vi "Partie 1.vi"() -> ()   [LabVIEW 2020]
uses:
  <instrlib>/Agilent 34401/Public/Data/Read (Multiple Points).vi
  <instrlib>/Agilent 2000 3000 X-Series/Public/Data/Read Measurement (Current Value).vi
  <instrlib>/Agilent 34401/Agilent 34401.lvlib
  <instrlib>/Agilent 2000 3000 X-Series/Agilent 2000 3000 X-Series.lvlib
panel:
  out "Nom du fichier":string
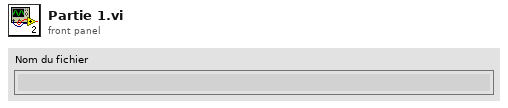
[diagram p1: front panel]
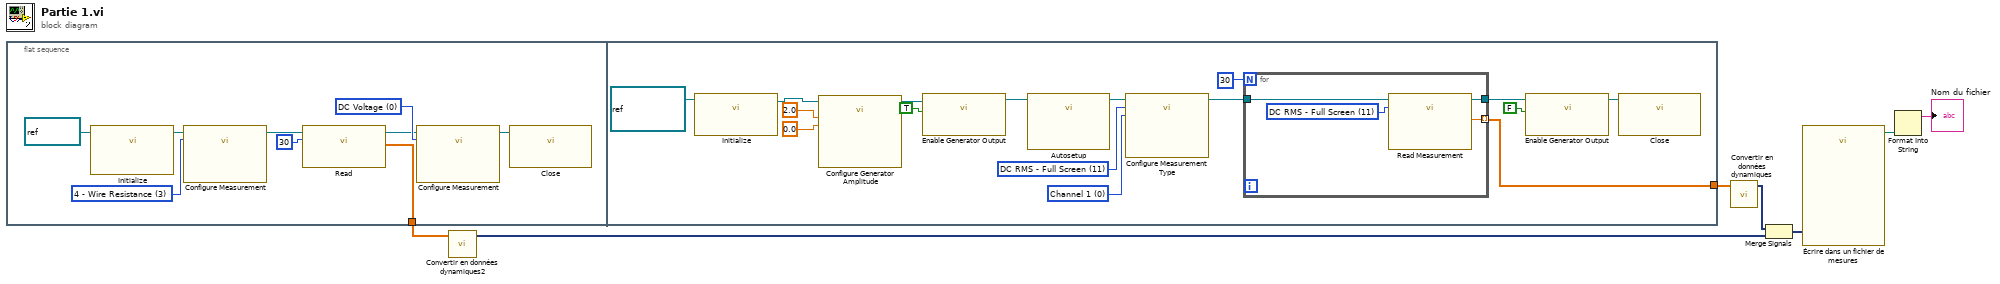
[diagram p0: block diagram]
diagram:
  n1 = flat-sequence {
    tunnel: [w10] -> w4
    tunnel: [w22] -> w7
    frame #0 {
      w16 = u16 0 items=["DC Voltage", "AC Voltage", "2 - Wire Resistance", "4 - Wire Resistance", "DC Current", "AC Current", "Frequency", "Period", "Continuity", "Diode Checking", "VDC:VDC Ratio", "Temperature", "Capacitance"] ("Function (0: DC Voltage)")
      w14 = u16 3 items=["DC Voltage", "AC Voltage", "2 - Wire Resistance", "4 - Wire Resistance", "DC Current", "AC Current", "Frequency", "Period", "Continuity", "Diode Checking", "VDC:VDC Ratio", "Temperature", "Capacitance"] ("Function (0: DC Voltage)")
      n2 = call <instrlib>:"Initialize.vi"("VISA resource name"=refnum<visa-resource-name> "GPIB0::22::INSTR") -> ("VISA resource name out"=w8:refnum<visa-resource-name>)  [unwired: 9 in, 1 out]
      n3 = call <instrlib>:"Configure Measurement.vi"("Function (0: DC Voltage)"=w14, "VISA resource name"=w8) -> ("VISA resource name out"=w13:refnum<visa-resource-name>)  [unwired: 8 in, 1 out]
      n4 = call-poly <instrlib>:"Read.vi"("Sample Count (1)"=30, "VISA resource name"=w13) -> ("Measurements"=w10:dbl[], "VISA resource name out"=w12:refnum<visa-resource-name>)  [unwired: 7 in, 1 out]
      n5 = call <instrlib>:"Configure Measurement.vi"("Function (0: DC Voltage)"=w16, "VISA resource name"=w12) -> ("VISA resource name out"=w9:refnum<visa-resource-name>)  [unwired: 8 in, 1 out]
      n6 = call <instrlib>:"Close.vi"("VISA resource name"=w9) -> ()  [unwired: 10 in, 1 out]
    }
    frame #1 {
      w29 = 0 items=["Channel 1"=0, "Channel 2"=1, "Channel 3"=2, "Channel 4"=3, "Waveform Memory 1"=5, "Waveform Memory 2"=6, "Serial Bus 1"=7, "Serial Bus 2"=8, "Digital Bus Low"=9, "Digital Bus High "=10, "Digital Bus 1"=11, "Digital Bus 2"=12, "D0"=13, "D1"=14, "D2"=15, "D3"=16, "D4"=17, "D5"=18, "D6"=19, "D7"=20, "D8"=21, "D9"=22, "D10"=23, "D11"=24, "D12"=25, "D13"=26, "D14"=27, "D15"=28, "External"=29, "Function 1"=32, "Function 2"=33, "Function 3"=34, "Function 4"=35, "Math 1"=36, "Math 2"=37, "Math 3"=38, "Math 4"=39, "FFT"=40, "Analog Bus"=41] ("Measurement Source 1 (0: Channel 1)")
      w30 = 11 items=["Peak-Peak", "Maximum", "Minimum", "Amplitude", "Top", "Base", "Overshoot", "Preshoot", "Average - N Cycles", "Average - Full Screen", "DC RMS - N Cycles", "DC RMS - Full Screen", "AC RMS - N Cycles", "AC RMS - Full Screen (Std Dev)", "Ratio", "Period", "Frequency", "Counter", "+Width", "-Width", "Burst Width", "Duty Cycle", "Rise Time", "Fall Time", "Delay", "Phase", "X minY", "X maxY", "Positive Pulse Count", "Negative Pulse Count", "Raising Edge Count", "Falling Edge Count", "Area - N Cycle", "Area - Full Screen", "Bit Rate", "Negative Duty Cycle", "Standard Deviation"] ("Measurement Type (0: Peak-Peak)")
      n7 = call <instrlib>:"Initialize.vi"("VISA resource name"=refnum<visa-resource-name> "GPIB0::7::INSTR") -> ("VISA resource name out"=w18:refnum<visa-resource-name>)  [unwired: 9 in, 1 out]
      n8 = call <instrlib>:"Configure Generator Amplitude.vi"("VISA resource name"=w18, "Amplitude (1.0 V)"=2.0, "Offset (0.0 V)"=0.0) -> ("VISA resource name out"=w17:refnum<visa-resource-name>)  [unwired: 11 in, 1 out]
      n9 = call <instrlib>:"Enable Generator Output.vi"("Enable Output (F: Disable)"=TRUE, "VISA resource name"=w17) -> ("VISA resource name out"=w31:refnum<visa-resource-name>)  [unwired: 8 in, 1 out]
      n10 = call <instrlib>:"Autosetup.vi"("VISA resource name"=w31) -> ("VISA resource name out"=w28:refnum<visa-resource-name>)  [unwired: 9 in, 1 out]
      n11 = call <instrlib>:"Configure Measurement Type.vi"("VISA resource name"=w28, "Measurement Type (0: Peak-Peak)"=w30, "Measurement Source 1 (0: Channel 1)"=w29) -> ("VISA resource name out"=w26:refnum<visa-resource-name>)  [unwired: 11 in, 1 out]
      n12 = for {
        N: 30 -> [_]
        tunnel: w26 -> [w35]
        tunnel: [w34] -> w25
        tunnel: [w33] -> w22 mode=indexing
        w36 = 11 items=["Peak-Peak", "Maximum", "Minimum", "Amplitude", "Top", "Base", "Overshoot", "Preshoot", "Average - N Cycles", "Average - Full Screen", "DC RMS - N Cycles", "DC RMS - Full Screen", "AC RMS - N Cycles", "AC RMS - Full Screen (Std Dev)", "Ratio", "Period", "Frequency", "Counter", "+Width", "-Width", "Burst Width", "Duty Cycle", "Rise Time", "Fall Time", "Delay", "Phase", "X minY", "X maxY", "Positive Pulse Count", "Negative Pulse Count", "Raising Edge Count", "Falling Edge Count", "Area - N Cycle", "Area - Full Screen", "Nth Edge Time", "Nth Edge Cross Level Time", "Bit Rate", "Negative Duty Cycle", "Standard Deviation"] ("Measurement Type (0: Peak-Peak)")
        n13 = call-poly <instrlib>:"Read Measurement.vi"("VISA resource name"=w35, "Measurement Type (0: Peak-Peak)"=w36) -> ("VISA resource name out"=w34:refnum<visa-resource-name>, "Result Value"=w33:dbl)  [unwired: 11 in, 1 out]
      }
      n14 = call <instrlib>:"Enable Generator Output.vi"("Enable Output (F: Disable)"=FALSE, "VISA resource name"=w25) -> ("VISA resource name out"=w23:refnum<visa-resource-name>)  [unwired: 8 in, 1 out]
      n15 = call <instrlib>:"Close.vi"("VISA resource name"=w23) -> ()  [unwired: 10 in, 1 out]
    }
  }
  n16 = call "Convertir en données dynamiques2"("Array"=w4) -> ("Dynamic Data Type"=w3:dynamicdata)  [unwired: 3 in]
  n17 = call "Convertir en données dynamiques"("Array"=w7) -> ("Dynamic Data Type"=w6:dynamicdata)  [unwired: 3 in]
  n18 = Merge Signals(w6, w3) -> (w5:dynamicdata)
  n19 = call "Écrire dans un fichier de mesures"("Signals"=w5) -> ("Filename Out"=w2:path)  [unwired: 16 in, 2 out]
  n20 = Format Into String(w2) -> (resulting string=→"Nom du fichier":string)  [unwired: 3 in, 1 out]
